vi "New Results (to override).vi"(7 "Image Nr.":i32, 8 "error in (no error)":errorcluster, 9 "Results In":refnum<class "Analyze Results Base.lvclass">[](array[class]), 10 "Parameters":refnum<class "Analyze Parameter Base.lvclass">[](array[class]), 11 "Launch IMAQ Display in":refnum<class "HIJ File Viewer Demo App.lvclass">) -> (0 "error out":errorcluster, 3 "Launch IMAQ Display out":refnum<class "HIJ File Viewer Demo App.lvclass">)   [LabVIEW 2014, in "HIJ File Viewer Demo App.lvlib" / "HIJ File Viewer Demo App.lvclass"]
uses:
  HIJ File Viewer Demo App.lvclass
  Analyze/Results and Overlays/Results Base/Analyze Results Base.lvclass
  Analyze/Analyze Parameter/Analyze Parameter Base/Analyze Parameter Base.lvclass
  Application Base Actors/HIJ Vision File Viewer App/HIJ Vision File Viewer App/HIJ Vision File Viewer App.lvclass
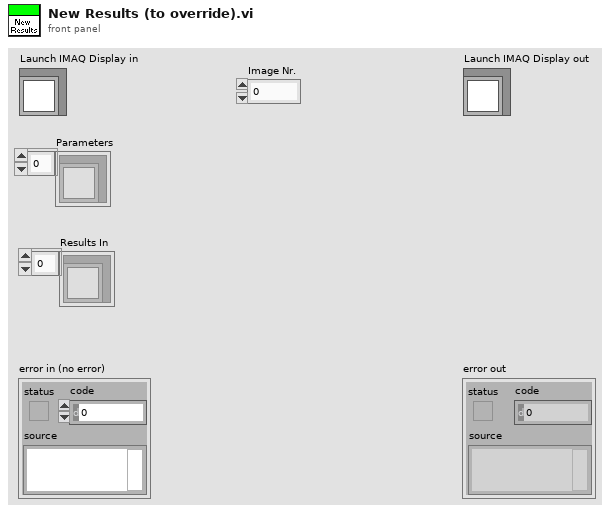
[diagram p1: front panel]
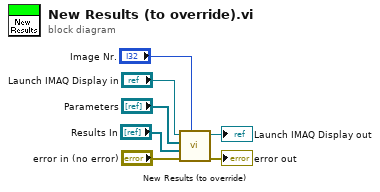
[diagram p0: block diagram]
diagram:
  n1 = call-parent "New Results (to override).vi"("Image Nr."="Image Nr.", "error in (no error)"="error in (no error)", "Results In"="Results In", "Parameters"="Parameters", "Launch IMAQ Display in"="Launch IMAQ Display in") -> ("error out"=→"error out":errorcluster, "Launch IMAQ Display out"=→"Launch IMAQ Display out":refnum<class "HIJ File Viewer Demo App.lvclass">)  [unwired: 5 in]
